vi "Configure Bitfile.vi"(0 "USRP RIO device":T1, 5 "which bitfile":string(combo)="Time", 11 "error in":errorcluster) -> (4 "USRP RIO device":T1, 6 "bitfile":path, 15 "error out":errorcluster)   [LabVIEW 2020]
uses:
  <vilib>/userdefined/Silver/nirio_resource_slv.ctl
  <vilib>/Utility/error.llb/Error Cluster From Error Code.vi
  <vilib>/regexp/Match Regular Expression.xnode
  <vilib>/ErrorRing/Error Ring.xnode
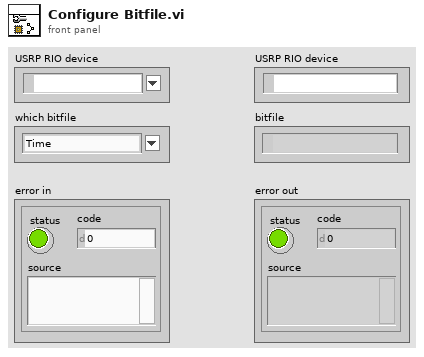
[diagram p1: front panel]
types:
  T1 = typedef "nirio_resource_slv.ctl" = tag
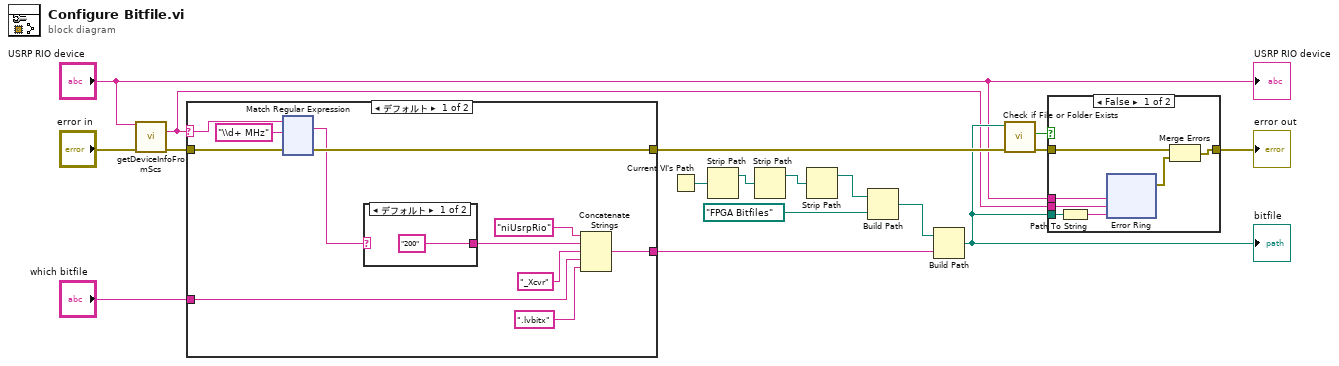
[diagram p0: block diagram]
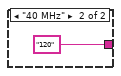
[diagram p3: hidden frame]
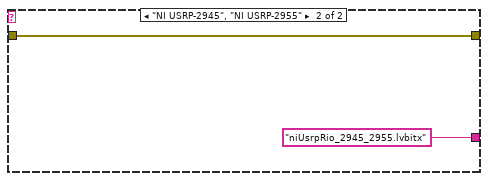
[diagram p4: hidden frame]
diagram:
  n1 = call <vilib>:"getDeviceInfoFromScs.vi"("rio device"="USRP RIO device", "error in"="error in") -> ("product name"=w5:string, "error out"=w9:errorcluster)  [unwired: 9 in, 3 out]
  n2 = case shown="デフォルト" w5 {
    selector: w5 -> [w18 _]
    tunnel: "which bitfile" -> [w25 _]
    tunnel: w9 -> [w23 w145]
    tunnel: [w22 w145] -> w7
    tunnel: [w19 "niUsrpRio_2945_2955.lvbitx" ("f")] -> w8
    frame Default {
      n3 = xnode "Match Regular Expression"("input string"=w18, "regular expression"="\\d+ MHz", "error in"=w23) -> ("whole match"=w21:string, "error out"=w22:errorcluster)  [unwired: 3 in, 3 out]
      n4 = case shown="デフォルト" w21 {
        tunnel: ["200" ("format string") "120" ("format string")] -> w20
        frame Default {
        }
        frame "40 MHz" {
        }
      }
      n5 = Concatenate Strings("niUsrpRio" ("format string"), w20, "_Xcvr" ("format string"), w25, ".lvbitx" ("format string")) -> (w19:string)
    }
    frame "NI USRP-2945", "NI USRP-2955" {
    }
  }
  n6 = Current VI's Path() -> (path=w17:path)
  n7 = Strip Path(path=w17) -> (stripped path=w14:path)  [unwired: 1 out]
  n8 = Strip Path(path=w14) -> (stripped path=w13:path)  [unwired: 1 out]
  n9 = Strip Path(path=w13) -> (stripped path=w12:path)  [unwired: 1 out]
  n10 = Build Path(base path=w12, name or relative path=path "FPGA Bitfiles") -> (appended path=w15:path)
  n11 = Build Path(base path=w15, name or relative path=w8) -> (appended path=w6:path)
  "bitfile" <- w6
  n12 = call <vilib>:"Check if File or Folder Exists.vi"("error in (no error)"=w7, "path"=w6) -> ("error out"=w2:errorcluster, "file or folder exists?"=w1:bool)  [unwired: 7 in, 1 out]
  n13 = case shown="FALSE" w1 {
    tunnel: w6 -> [w153 _]
    tunnel: w5 -> [w151 _]
    tunnel: "USRP RIO device" -> [w150 _]
    tunnel: [w148 w163] -> w3
    tunnel: w2 -> [w149 w163]
    frame False {
      n14 = Path To String(path=w153) -> (string=w152:string)
      n15 = xnode "Error Ring"("パラメータ 0"=w150, "パラメータ 1"=w151, "パラメータ 2"=w152) -> ("エラー出力"=w147:errorcluster)
      n16 = Merge Errors(w149, w147) -> (w148:errorcluster)
    }
    frame True {
    }
  }
  "error out" <- w3
  "USRP RIO device" <- "USRP RIO device"
